vi "dataset.rid.vi"(8 "error in":errorcluster, 11 "Dataset in":refnum<class "Dataset.lvclass">) -> (0 "error out":errorcluster, 2 "rid":string, 3 "Dataset out":refnum<class "Dataset.lvclass">)   [LabVIEW 2020, in "Dataset.lvclass"]
doc: "Returns the dataset's RID."
uses:
  Dataset.lvclass
  Dataset.lvclass/Dataset.ctl
  client.lvlib
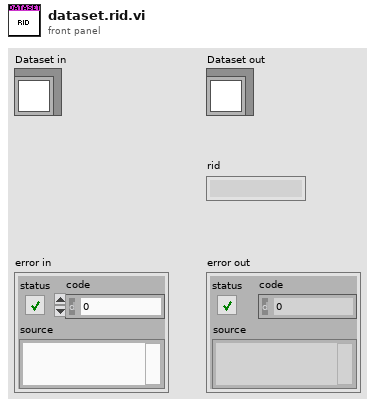
[diagram p1: front panel]
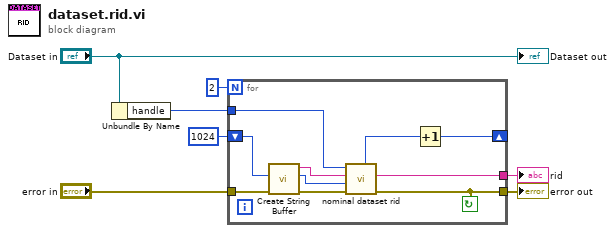
[diagram p0: block diagram]
diagram:
  n1 = Unbundle By Name("Dataset in") -> ("handle"=w4:i32)
  n2 = for {
    N: 2 -> [_]
    tunnel: w4 -> [w17]
    tunnel: [w16] -> w1
    shift-right: [w9] -> _
    shift-left: 1024 ("Buffer Size (1024)") -> [w13]
    tunnel: [w10] -> w3
    tunnel: "error in" -> [w8]
    stop <- w10 continue-if-true
    n3 = call "Create String Buffer.vi"("error in"=w8, "Buffer Size (1024)"=w13) -> ("error out"=w12:errorcluster, "dub Buffer Size"=w14:i32, "String Buffer"=w15:string)  [unwired: 7 in]
    n4 = call "nominal dataset rid.vi"("error in (no error)"=w12, "cap"=w14, "buf"=w15, "dataset"=w17) -> ("error out"=w10:errorcluster, "buf out"=w16:string, "out_needed out"=w11:u32)  [unwired: 4 in, 1 out]
    n5 = Increment(x=w11) -> (x+1=w9:u32)
  }
  "error out" <- w3
  "rid" <- w1
  "Dataset out" <- "Dataset in"
